vi "Register Channel.vi"(8 "error in (no error)":errorcluster, 9 "Channel":refnum<class "CIFChannels.lvclass">, 11 "CIFChannelMng in":refnum<class "CIFChannelMng.lvclass">) -> (0 "error out":errorcluster, 3 "CIFChannelMng out":refnum<class "CIFChannelMng.lvclass">)   [LabVIEW 2021, in "CIFChannelMng.lvclass"]
uses:
  CIFChannelMng.lvclass
  CIFChannels/CIFChannels.lvclass
  CIFChannels/CIFChannels.lvclass/CIFChannels.ctl
  CIFClocks/Typedef/Errors.ctl
  CIFChannelMng.lvclass/CIFChannelMng.ctl
  CIFCore/Common/Utilities/Append Error Location.vi
  CIFCore/Common/CIFCoreCommon.lvlib
  CIFChannels/Typedef/Direction.ctl
  typedef/Channel List for OOB.ctl
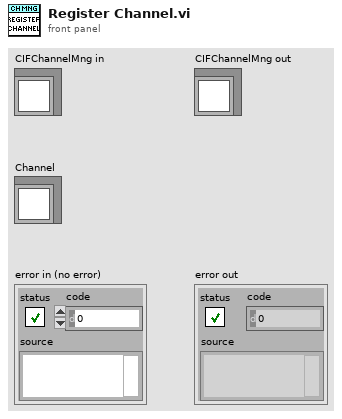
[diagram p1: front panel]
types:
  T1 = typedef "CIFCoreCommon.lvlib/Errors.ctl" = enum16{"Invalid Clock ID", "Long Sleep", "gRPC Server Not Found", "Config Parse", "Timestamp Wrap", "Delayed Execution", "Duplicate Channel", "Missing Channel", "Incorrect Type", "Unregistered Enum"}
  T2 = typedef "CIFChannels.lvclass/Direction.ctl" = enum16{"Publisher", "Subscriber"}
  T3 = typedef "CIFChannelMng.lvclass/Channel List for OOB.ctl" = cluster{"Direction":T2, "Type":string, "Custom Config Data":variant, "Connected?":bool, "Connected Name":string}
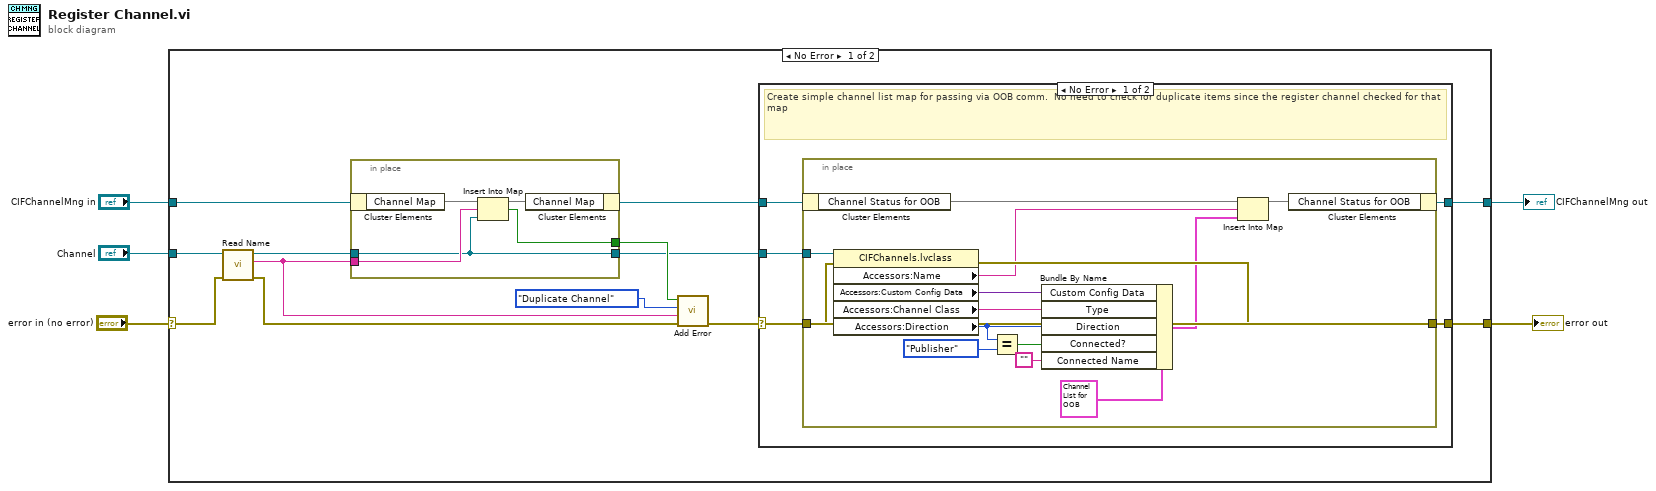
[diagram p0: block diagram]
diagram:
  n1 = case shown="No Error" "error in (no error)" {
    selector: "error in (no error)" -> [w13 w45]
    tunnel: [w9 w45] -> w4
    tunnel: [w6 w44] -> w2
    tunnel: "CIFChannelMng in" -> [w17 w44]
    tunnel: "Channel" -> [w14 _]
    frame No Error {
      n2 = call "Read Name.vi"("error in (no error)"=w13, "CIFChannels in"=w14) -> ("error out"=w12:errorcluster, "Name"=w10:string, "CIFChannels out"=w11:refnum<class "CIFChannels.lvclass">)  [unwired: 7 in]
      n3 = in-place {
        in-place-border: w10 -> [w41]
        in-place-border: w11 -> [w39]
        in-place-border: [w40] -> w16
        in-place-border: [w39] -> w7
        n4 = in-place-cluster #1(w17) -> ("Channel Map"=w43:map{string, refnum<class "CIFChannels.lvclass">})
        n5 = Insert Into Map(map in=w43, key=w41, value=w39) -> (map out=w42:map{string, refnum<class "CIFChannels.lvclass">}, key already included?=w40:bool)  [unwired: 1 out]
        n6 = in-place-cluster #1("Channel Map"=w42) -> (w8:refnum<class "CIFChannelMng.lvclass">)
      }
      n7 = call "Add Error.vi"("error in (no error)"=w12, "String to Append"=w10, "Error"=Errors."Duplicate Channel", "Insert Error"=w16) -> ("error out"=w9:errorcluster)  [unwired: 7 in]
      n8 = case shown="No Error" w9 {
        selector: w9 -> [w19 w37]
        tunnel: w8 -> [w22 w38]
        tunnel: w7 -> [w21 _]
        tunnel: [w20 w38] -> w6
        tunnel: [w18 w37] -> _
        frame No Error {
          # "Create simple channel list map for passing via OOB comm.  No need to check for duplicate items since the register channel checked for that map"
          n9 = in-place {
            in-place-border: w21 -> [w36]
            in-place-border: w19 -> [w32]
            in-place-border: [w31] -> w18
            n10 = in-place-cluster #2(w22) -> ("Channel Status for OOB"=w30:map{string, T3})
            n11 = property class="CIFChannels.lvclass"(reference=w36, error in=w32) -> (error out=w31:errorcluster, "Accessors:Name"=w27:string, "Accessors:Custom Config Data"=w33:variant, "Accessors:Channel Class"=w34:string, "Accessors:Direction"=w25:T2)  [unwired: 1 out]
            n12 = Equal?(x=w25, y=Direction."Publisher") -> (x = y?=w23:bool)
            n13 = Bundle By Name(cluster=T3 {"Direction"=enum."Publisher", "Type"="", "Custom Config Data"=variant, "Connected?"=FALSE, "Connected Name"=""} ("Channel List"), "Custom Config Data"=w33, "Type"=w34, "Direction"=w25, "Connected?"=w23, "Connected Name"="") -> (w28:T3)
            n14 = Insert Into Map(map in=w30, key=w27, value=w28) -> (map out=w29:map{string, T3})  [unwired: 2 out]
            n15 = in-place-cluster #2("Channel Status for OOB"=w29) -> (w20:refnum<class "CIFChannelMng.lvclass">)
          }
        }
        frame Error {
        }
      }
    }
    frame Error {
    }
  }
  "error out" <- w4
  "CIFChannelMng out" <- w2
